vi "Washer DOE Shutdown Global.vi"() -> ()   [LabVIEW 2014]
uses:
  DOE Global Control.ctl
panel:
  out "ZM301 Global":T1
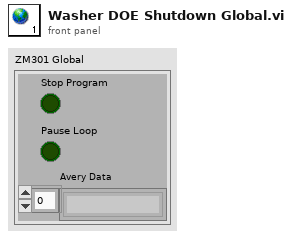
[diagram p1: front panel]
types:
  T1 = typedef "DOE Global Control.ctl" = cluster{"Stop Program":bool, "Pause Loop":bool, "Avery Data":string[]}
diagram:
